vi "From JSON.vi"(8 "error in (no error)":errorcluster, 10 "JSON Config":path, 11 "object in":refnum<class "Configuration Base.lvclass">) -> (0 "error out":errorcluster, 3 "object out":refnum<class "Configuration Base.lvclass">)   [LabVIEW 2023, in "HAL.lvlib" / "Configuration Base.lvlib" / "Configuration Base.lvclass"]
uses:
  Configuration Base.lvclass
  Configuration Base.lvclass/Configuration Base.ctl
  <vilib>/Utility/error.llb/Error Cluster From Error Code.vi
  <vilib>/ErrorRing/Error Ring.xnode
  <vilib>/JDP Science/JSONtext/Config Files/Config File.lvclass
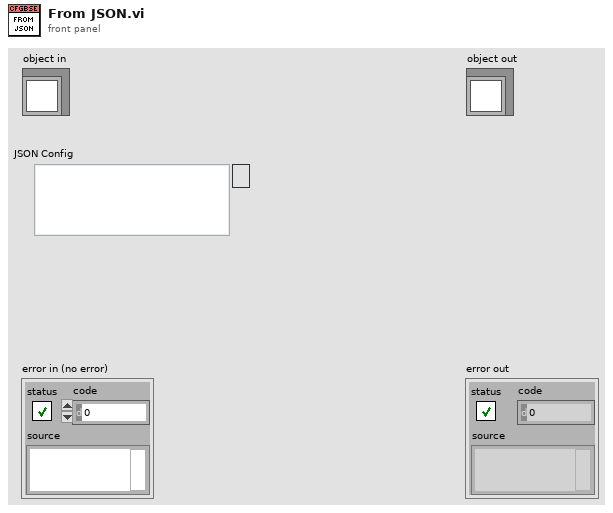
[diagram p1: front panel]
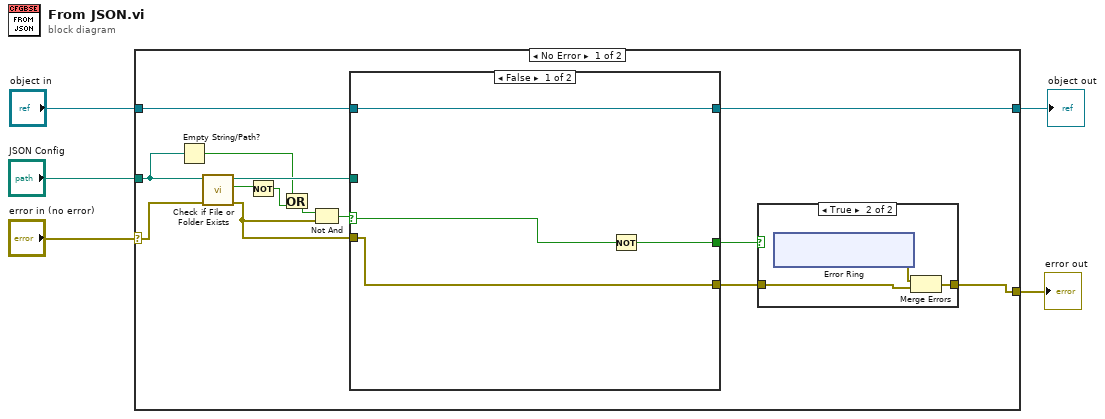
[diagram p0: block diagram]
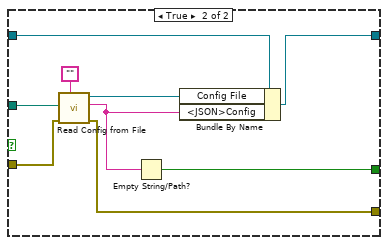
[diagram p3: hidden frame]
diagram:
  n1 = case shown="No Error" "error in (no error)" {
    selector: "error in (no error)" -> [w15 w43]
    tunnel: [w6 w43] -> w4
    tunnel: [w14 w42] -> w2
    tunnel: "object in" -> [w16 w42]
    tunnel: "JSON Config" -> [w13 _]
    frame No Error {
      n2 = Empty String/Path?(string/path=w13) -> (empty?=w12:bool)
      n3 = call <vilib>:"Check if File or Folder Exists.vi"("error in (no error)"=w15, "path"=w13) -> ("error out"=w18:errorcluster, "file or folder exists?"=w17:bool, "dup path"=w19:path)  [unwired: 7 in]
      n4 = Not(x=w17) -> (.not. x?=w11:bool)
      n5 = Or(x=w12, y=w11) -> (x .or. y?=w10:bool)
      n6 = Not And(1:w18, 2:w10) -> (0:w9:bool)
      n7 = case shown="False" w9 {
        selector: w9 -> [w31 _]
        tunnel: w16 -> [w32 w39]
        tunnel: [w32 w37] -> w14
        tunnel: w19 -> [_ w41]
        tunnel: w18 -> [w29 w40]
        tunnel: [w30 w34] -> w8
        tunnel: [w29 w33] -> w7
        frame False {
          n8 = Not(x=w31) -> (.not. x?=w30:bool)
        }
        frame True {
          n9 = call <vilib>:"Read Config from File.vi"("Template (JSON Object)"="", "error in (no error)"=w40, "config file path"=w41) -> ("error out"=w33:errorcluster, "<JSON>Config"=w35:string, "Config File"=w38:refnum<class "Config File.lvclass">)  [unwired: 5 in, 1 out]
          n10 = Empty String/Path?(string/path=w35) -> (empty?=w34:bool)
          n11 = Bundle By Name(cluster=w39, "Config File"=w38, "<JSON>Config"=w35) -> (w37:refnum<class "Configuration Base.lvclass">)
        }
      }
      n12 = case shown="True" w8 {
        tunnel: w7 -> [w20 w21]
        tunnel: [w20 w23] -> w6
        frame False {
        }
        frame True {
          n13 = xnode "Error Ring"() -> ("error out"=w22:errorcluster)
          n14 = Merge Errors(w22, w21) -> (w23:errorcluster)
        }
      }
    }
    frame Error {
    }
  }
  "error out" <- w4
  "object out" <- w2
